vi "test_Find peaks.vi"() -> ()   [LabVIEW 2014]
uses:
  Melody Extraction.lvlib
panel:
  out "Waveform Graph":dbl[](graph)
  out "Intensity Graph":dbl[][](graph)
  out "Peak Magnitudes":dbl[](array[numeric])
  out "Peaks Frequencies":dbl[](array[numeric])
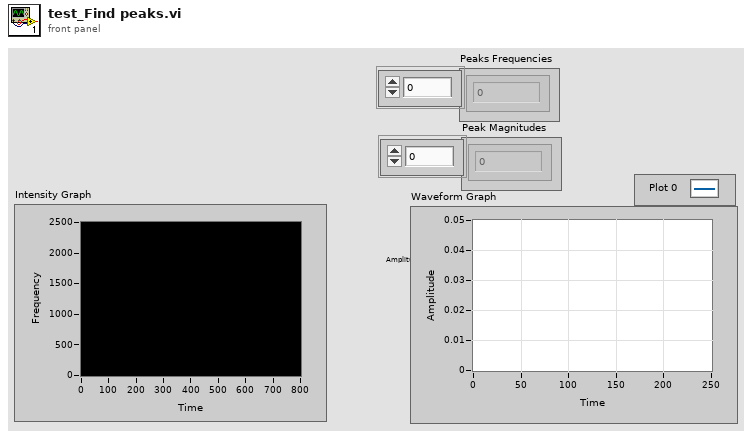
[diagram p1: front panel]
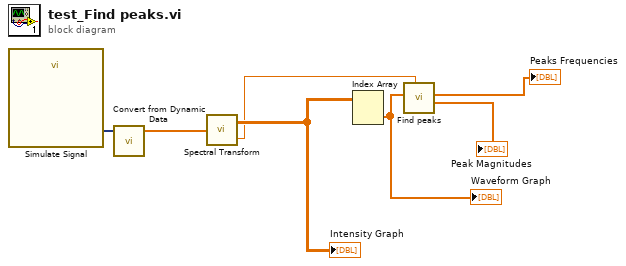
[diagram p0: block diagram]
diagram:
  n1 = call "Simulate Signal"() -> ("Sine"=w7:dynamicdata)  [unwired: 14 in, 1 out]
  n2 = call "Convert from Dynamic Data"("Dynamic Data Type"=w7) -> ("Array"=w4:dbl[])  [unwired: 3 in]
  n3 = call "Spectral Transform.vi"("Input Signal"=w4) -> ("STFT"=w3:dbl[][], "Frequency Axis Scale Factor"=w1:dbl)
  "Intensity Graph" <- w3
  n4 = Index Array(array=w3) -> (element=w5:dbl[])  [unwired: 2 in]
  "Waveform Graph" <- w5
  n5 = call "Find peaks.vi"("Frequency Axis Scale Factor"=w1, "FFT (single frame)"=w5) -> ("Peak Magnitudes"=→"Peak Magnitudes":dbl[], "Peaks Frequencies"=→"Peaks Frequencies":dbl[])  [unwired: 8 in]
